vi "FTW-JSON-Parse.vi"(5 "JSON String":string, 11 "error in":errorcluster) -> (4 "Container":refnum<class "FTW-Container.lvclass">, 15 "error out":errorcluster)   [LabVIEW 2015]
uses:
  container/FTW-Container.lvclass
  FTW-JSON-LexicalScan.ctl
panel:
  # "Inputs"
  # "Outputs"
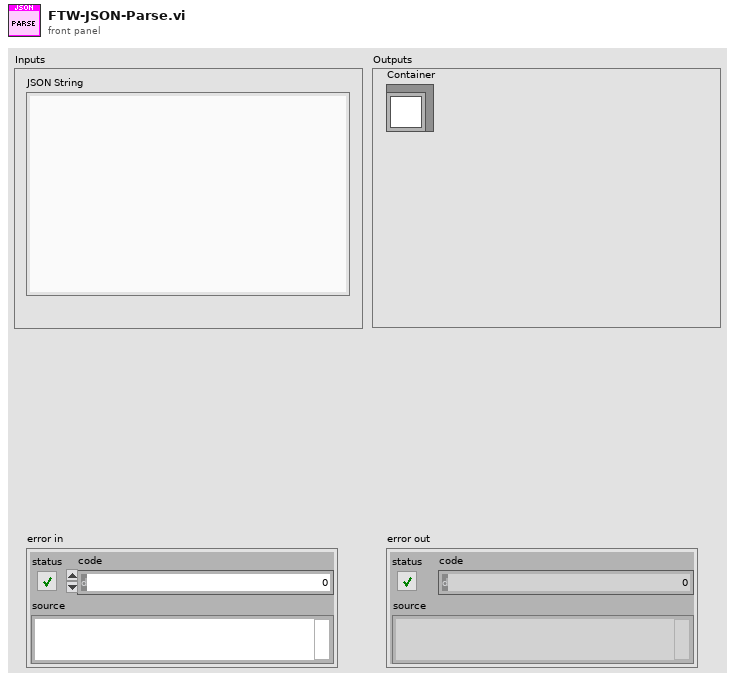
[diagram p1: front panel]
types:
  T1 = typedef "FTW-JSON-LexicalScan.ctl" = cluster{"String":string, "Position":i32, "Line":i32, "Column":i32, "Last Column":i32}
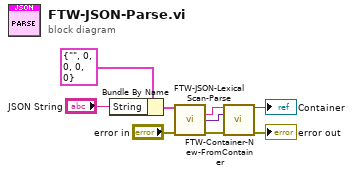
[diagram p0: block diagram]
diagram:
  n1 = Bundle By Name(cluster=T1 {"String"="", "Position"=0, "Line"=0, "Column"=0, "Last Column"=0} ("JSON String"), "String"="JSON String") -> (w2:T1)
  n2 = call "FTW-JSON-LexicalScan-Parse.vi"("JSON String"=w2, "error in"="error in") -> ("Name"=w6:string, "Container"=w5:variant, "error out"=w9:errorcluster)  [unwired: 10 in, 1 out]
  n3 = call "FTW-Container-New-FromContainer.vi"("Name"=w6, "Container"=w5, "error in"=w9) -> ("FTW-Container"=→"Container":refnum<class "FTW-Container.lvclass">, "error out"=→"error out":errorcluster)  [unwired: 11 in]
